vi "_prepareForW&R_EEPROM_vna_wmg.vi"(4 "Select channel":u32 max=1, 5 "Mode":u32(ring) items=["0~EasyI2C", "1~TimingI2C"], 6 "VISA resource name":refnum<visa-resource-name>="COM1") -> (0 "错误输出":errorcluster, 1 "x = y?":bool, 2 "VISA资源名称输出":refnum<visa-resource-name>)   [LabVIEW 2011]
uses:
  <vilib>/Instr/_visa.llb/VISA Configure Serial Port (Instr).vi
panel:
  in  "Error in":errorcluster
  # "Input"
  # "Output"
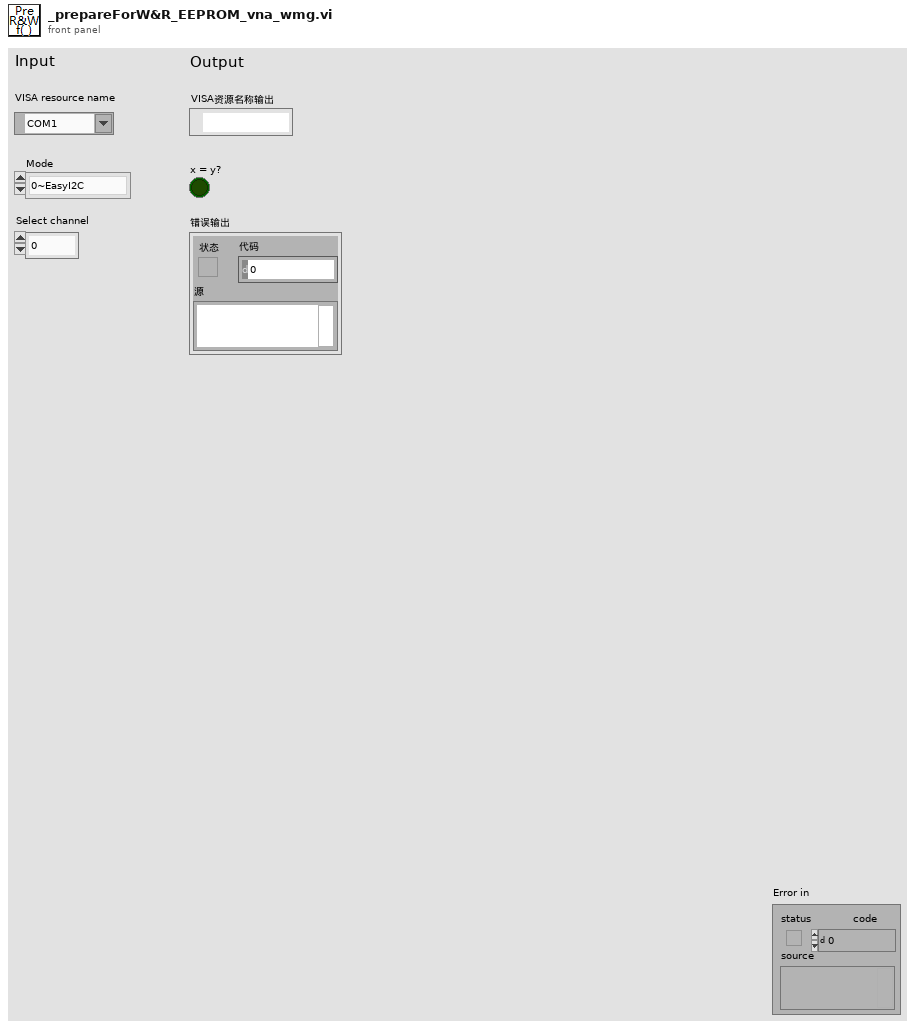
[diagram p1: front panel]
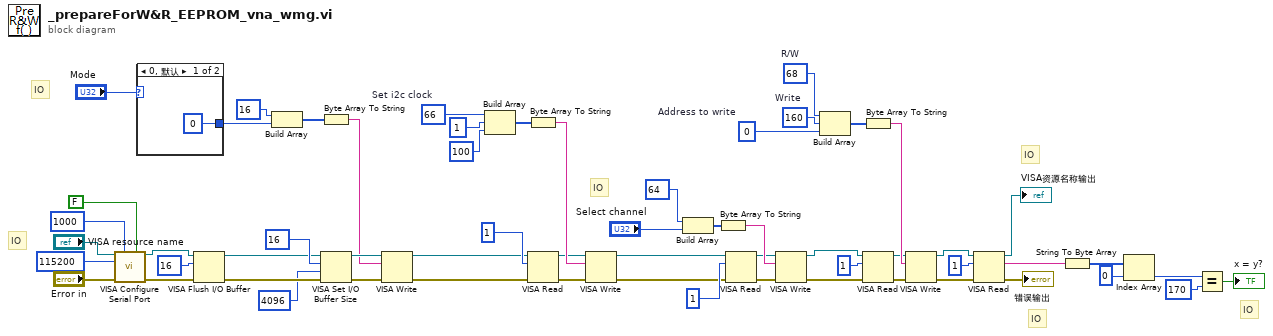
[diagram p0: block diagram]
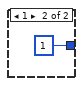
[diagram p2: hidden frame]
diagram:
  w24 = u32 0  # Address to write
  w28 = u32 160  # Write
  w26 = u32 68  # R/W
  w41 = u32 66  # Set i2c clock
  # "IO"
  # "IO"
  # "IO"
  # "IO"
  # "IO"
  # "IO"
  n1 = call-poly "VISA Configure Serial Port"("VISA resource name"="VISA resource name", "timeout (10sec)"=u32 1000 ("timeout"), "Enable Termination\nChar (T)"=FALSE ("Enable Termination\nChar (T)"), "baud rate (9600)"=u32 115200 ("baud rate"), "error in (no error)"="Error in") -> ("VISA resource name out"=w59:refnum<visa-resource-name>, "error out"=w34:errorcluster)  [unwired: 9 in]
  n2 = case shown="0, 默认" "Mode" {
    tunnel: [u32 0 ("channel") u32 1 ("channel")] -> w47
    frame 0, Default {
    }
    frame 1 {
    }
  }
  n3 = VISA Flush I/O Buffer(VISA resource name=w59, mask (16)=u16 16, error in (no error)=w34) -> (VISA resource name out=w56:refnum<visa-resource-name>, error out=w55:errorcluster)
  n4 = Build Array(u32 16 ("size (0)"), w47) -> (w46:u32[])
  n5 = Byte Array To String(unsigned byte array=w46) -> (string=w49:string)
  n6 = VISA Set I/O Buffer Size(VISA resource name=w56, mask (16)=u16 16, size (4096)=u32 4096 ("size (0)"), error in (no error)=w55) -> (VISA resource name out=w50:refnum<visa-resource-name>, error out=w33:errorcluster)
  n7 = VISA Write(VISA resource name=w50, write buffer=w49, error in (no error)=w33) -> (VISA resource name out=w14:refnum<visa-resource-name>, error out=w13:errorcluster)  [unwired: 1 out]
  n8 = Build Array(w41, u32 1 ("size (0)"), u32 100 ("size (0)")) -> (w40:u32[])
  n9 = Byte Array To String(unsigned byte array=w40) -> (string=w36:string)
  n10 = VISA Read(VISA resource name=w14, byte count=u32 1, error in (no error)=w13) -> (VISA resource name out=w12:refnum<visa-resource-name>, error out=w9:errorcluster)  [unwired: 2 out]
  n11 = VISA Write(VISA resource name=w12, write buffer=w36, error in (no error)=w9) -> (VISA resource name out=w11:refnum<visa-resource-name>, error out=w8:errorcluster)  [unwired: 1 out]
  n12 = Build Array(u32 64 ("size (0)"), "Select channel") -> (w45:u32[])
  n13 = Byte Array To String(unsigned byte array=w45) -> (string=w37:string)
  n14 = VISA Read(VISA resource name=w11, byte count=u32 1, error in (no error)=w8) -> (VISA resource name out=w10:refnum<visa-resource-name>, error out=w7:errorcluster)  [unwired: 2 out]
  n15 = VISA Write(VISA resource name=w10, write buffer=w37, error in (no error)=w7) -> (VISA resource name out=w6:refnum<visa-resource-name>, error out=w5:errorcluster)  [unwired: 1 out]
  n16 = Build Array(w26, w28, w24) -> (w27:u32[])
  n17 = Byte Array To String(unsigned byte array=w27) -> (string=w31:string)
  n18 = VISA Read(VISA resource name=w6, byte count=u32 1, error in (no error)=w5) -> (VISA resource name out=w3:refnum<visa-resource-name>, error out=w2:errorcluster)  [unwired: 2 out]
  n19 = VISA Write(VISA resource name=w3, write buffer=w31, error in (no error)=w2) -> (VISA resource name out=w25:refnum<visa-resource-name>, error out=w32:errorcluster)  [unwired: 1 out]
  n20 = VISA Read(VISA resource name=w25, byte count=u32 1, error in (no error)=w32) -> (VISA resource name out=→"VISA资源名称输出":refnum<visa-resource-name>, read buffer=w30:string, error out=→"错误输出":errorcluster)  [unwired: 1 out]
  n21 = String To Byte Array(string=w30) -> (unsigned byte array=w21:u8[])
  n22 = Index Array(array=w21, index=0) -> (element=w23:u8)
  n23 = Equal?(x=w23, y=u32 170 ("size (0)")) -> (x = y?=→"x = y?":bool)
